vi "test.vi"() -> ()   [LabVIEW 2011, in "双模温度计.xctl"]
panel:
  in  "双模温度计 2":dbl=20.0
  out "双模温度计":dbl(xcontrol)
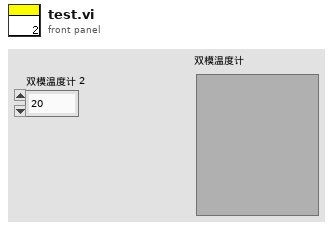
[diagram p1: front panel]
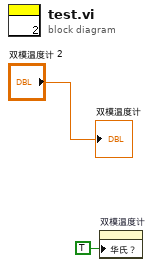
[diagram p0: block diagram]
diagram:
  n1 = property on="双模温度计" class="双模温度计 (strict)"("华氏？"=TRUE) -> ()  [unwired: 2 in, 2 out]
  "双模温度计" <- "双模温度计 2"
